vi "test Action Update Set Point-SetPoint30.vi"() -> ()   [LabVIEW 2018, in "AllComponentTestes.lvclass"]
uses:
  AllComponentTestes.lvclass
  C:/Program Files/National Instruments/LabVIEW 2018/vi.lib/addons/_JKI Toolkits/VI Tester/TestCase.llb/TestCase.lvclass
  <vilib>/addons/_JKI Toolkits/VI Tester/TestCase.llb/TestCase.lvclass
  Libraries/Thermal Chamber Controller_DQMH/Thermal Chamber Controller_DQMH.lvlib
panel:
  out "TestCase out":refnum<class "TestCase.lvclass">
  in  "TestCase in":refnum<class "AllComponentTestes.lvclass">
  out "error out":errorcluster
  in  "error in (no error)":errorcluster
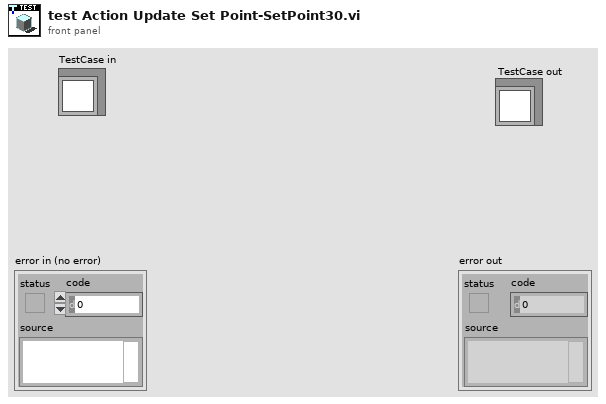
[diagram p1: front panel]
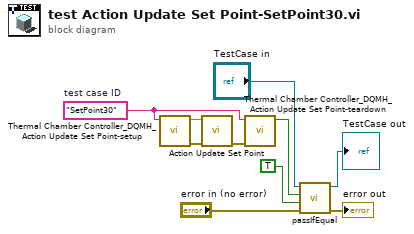
[diagram p0: block diagram]
diagram:
  w2 = "SetPoint30"  # test case ID
  n1 = call "Thermal Chamber Controller_DQMH_Action Update Set Point-setup.vi"("test case ID"=w2) -> ("error in"=w4:errorcluster, "Temperature Set Point"=w5:dbl)  [unwired: 9 in]
  n2 = call "Action Update Set Point.vi"("error in (no error)"=w4, "Temperature Set Point"=w5) -> ("error out"=w3:errorcluster)  [unwired: 9 in]
  n3 = call "Thermal Chamber Controller_DQMH_Action Update Set Point-teardown.vi"("error out"=w3, "test case ID"=w2) -> ("result"=w1:bool)  [unwired: 9 in]
  n4 = call-dynamic "passIfEqual.vi"("error in (no error)"="error in (no error)", "y"=TRUE, "x"=w1, "TestCase in"="TestCase in") -> ("error out"=→"error out":errorcluster, "TestCase out"=→"TestCase out":refnum<class "AllComponentTestes.lvclass">)  [unwired: 6 in]
